vi "GetSession Ref.vi"(8 "error in (no error)":errorcluster, 11 "Session in":refnum<class "Session.lvclass">) -> (0 "error out":errorcluster, 2 "Session Ref":refnum<k24>, 3 "Session out":refnum<class "Session.lvclass">)   [LabVIEW 2015, in "WinSCP.lvlib" / "Session.lvclass"]
uses:
  Session.lvclass
  C:/Users/Public/Documents/Projects/lv-winscp/Bin WinSCP/WinSCPnet.dll
  Bin WinSCP/WinSCPnet.dll
  Session.lvclass/Session.ctl
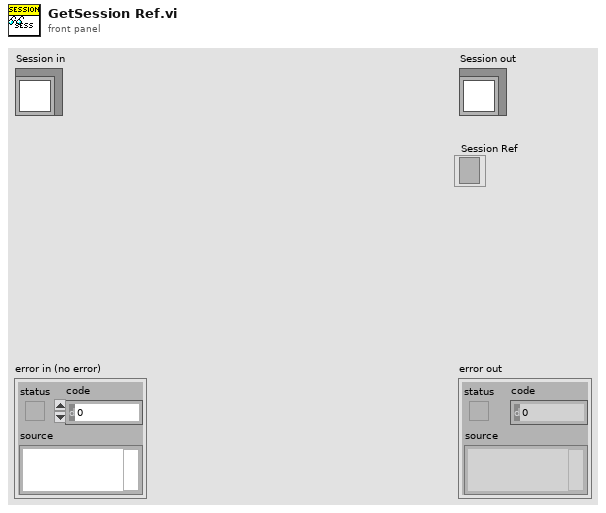
[diagram p1: front panel]
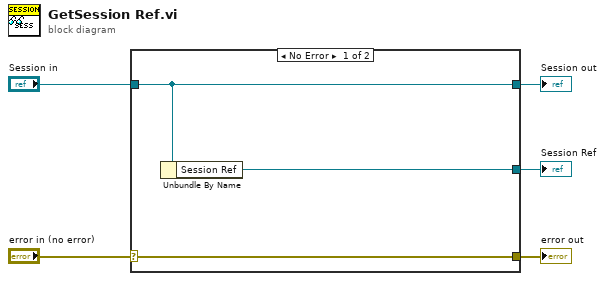
[diagram p0: block diagram]
diagram:
  n1 = case shown="No Error" "error in (no error)" {
    selector: "error in (no error)" -> [w8 w9]
    tunnel: [w8 w9] -> w4
    tunnel: [w7 w10] -> w2
    tunnel: "Session in" -> [w7 w10]
    tunnel: [w6 _] -> w1
    frame No Error {
      n2 = Unbundle By Name(w7) -> ("Session Ref"=w6:refnum<k24>)
    }
    frame Error {
    }
  }
  "error out" <- w4
  "Session out" <- w2
  "Session Ref" <- w1
